vi "Decide next action (rate-based).vi"(8 "error in (no error)":errorcluster, 9 "\"Good\" rate threshold":dbl, 10 "Seek positive polarization?":bool, 11 "Automatic Mode in":refnum<class "Automatic Mode.lvclass">) -> (0 "error out":errorcluster, 1 "New rate":dbl, 2 "Decision":T1, 3 "Automatic Mode out":refnum<class "Automatic Mode.lvclass">)   [LabVIEW 2015, in "Automatic Mode.lvclass"]
uses:
  Automatic Mode.lvclass
  Controller decision.ctl
  Automatic Mode.lvclass/Automatic Mode.ctl
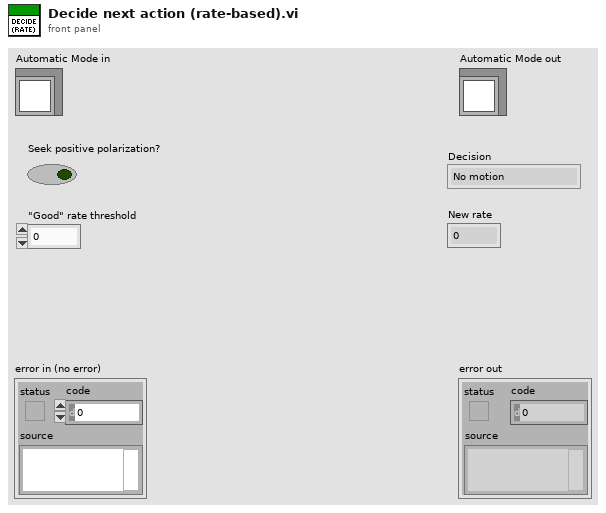
[diagram p1: front panel]
types:
  T1 = typedef "Controller decision.ctl" = enum16{"No motion", "Switch direction", "Keep current direction"}
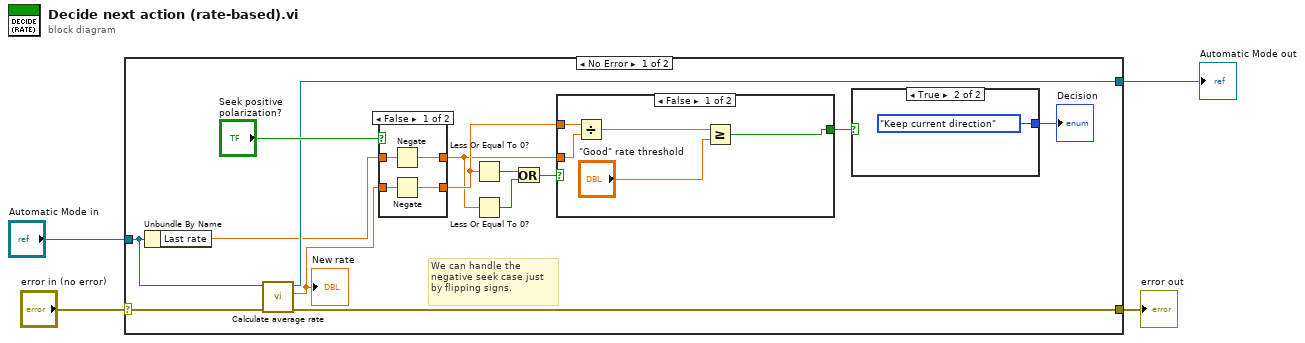
[diagram p0: block diagram]
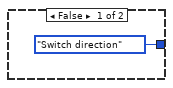
[diagram p2: hidden frame]
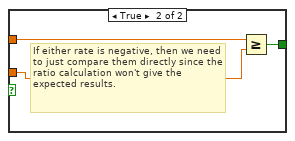
[diagram p3: hidden frame]
diagram:
  n1 = case shown="No Error" "error in (no error)" {
    selector: "error in (no error)" -> [w16 w36]
    tunnel: [w15 w36] -> w3
    tunnel: [w14 w35] -> w1
    tunnel: "Automatic Mode in" -> [w17 w35]
    frame No Error {
      # "We can handle the negative seek case just by flipping signs."
      n2 = Unbundle By Name(w17) -> ("Last rate"=w13:dbl)
      n3 = call "Calculate average rate.vi"("error in (no error)"=w16, "Automatic Mode in"=w17) -> ("error out"=w15:errorcluster, "Average rate"=w5:dbl, "Automatic Mode out"=w14:refnum<class "Automatic Mode.lvclass">)  [unwired: 7 in]
      "New rate" <- w5
      n4 = case shown="False" "Seek positive polarization?" {
        tunnel: w13 -> [w32 w33]
        tunnel: w5 -> [w31 w34]
        tunnel: [w30 w34] -> w9
        tunnel: [w29 w33] -> w8
        frame False {
          n5 = Negate(x=w32) -> (-x=w29:dbl)
          n6 = Negate(x=w31) -> (-x=w30:dbl)
        }
        frame True {
        }
      }
      n7 = Less Or Equal To 0?(x=w9) -> (x <= 0?=w12:bool)
      n8 = Less Or Equal To 0?(x=w8) -> (x <= 0?=w11:bool)
      n9 = Or(x=w12, y=w11) -> (x .or. y?=w10:bool)
      n10 = case shown="False" w10 {
        tunnel: w9 -> [w25 w28]
        tunnel: w8 -> [w24 w27]
        tunnel: [w21 w26] -> w7
        frame False {
          n11 = Divide(x=w25, y=w24) -> (x/y=w22:dbl)
          n12 = Greater Or Equal?(x=w22, y="\"Good\" rate threshold") -> (x >= y?=w21:bool)
        }
        frame True {
          # "If either rate is negative, then we need to just compare them directly since the ratio calculation won't give the expected results."
          n13 = Greater Or Equal?(x=w28, y=w27) -> (x >= y?=w26:bool)
        }
      }
      n14 = case shown="True" w7 {
        tunnel: [Controller_decision."Switch direction" ("Decision") Controller_decision."Keep current direction" ("Decision")] -> w6
        frame False {
        }
        frame True {
        }
      }
      "Decision" <- w6
    }
    frame Error {
    }
  }
  "error out" <- w3
  "Automatic Mode out" <- w1
